vi "Validate Configuration Metadata.vi"(8 "error in (no error)":errorcluster, 11 "MeasurementPluginService in":refnum<class "MeasurementPluginService.lvclass">) -> (0 "error out":errorcluster, 3 "MeasurementPluginService out":refnum<class "MeasurementPluginService.lvclass">)   [LabVIEW 2020, in "MeasurementLink Measurement Server.lvlib"]
uses:
  MeasurementLink Measurement Server.lvlib
  <vilib>/Utility/Data Type/NI_Data Type.lvlib
  Classes/MeasurementPluginService/MeasurementPluginService.lvclass
  Error Strings Global Internal.vi
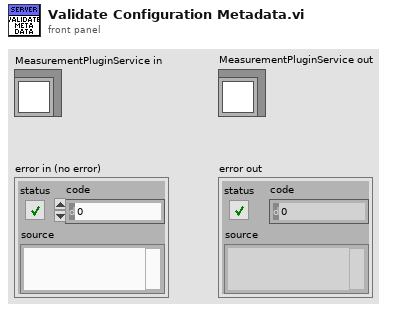
[diagram p1: front panel]
types:
  T1 = typedef "MeasurementLink Measurement Server.lvlib/MeasurementPluginService.lvclass/Plugin Paths.ctl" = cluster{"Get Measurement Details VI Path":path, "Get Type Specializations VI Path":path, "Get UI Details VI Path":path, "Measurement Logic VI Path":path, "Measurement Configuration CTL Path":path, "Measurement Results CTL Path":path}
  T2 = typedef "MeasurementLink Measurement Server.lvlib/Parameter Type Specialization.ctl" = cluster{"Parameter Name":string, "Type Specialization":T3, "Annotations":cluster{"Key":T4, "Value":string}[]}
  T3 = typedef "MeasurementLink Measurement Server.lvlib/Type Specialization.ctl" = enum16{"none", "pin", "path", "enum"}
  T4 = typedef "MeasurementLink Measurement Server.lvlib/Type Specialization Key.ctl" = enum16{"none", "pin.instrument_type", "enum.values"}
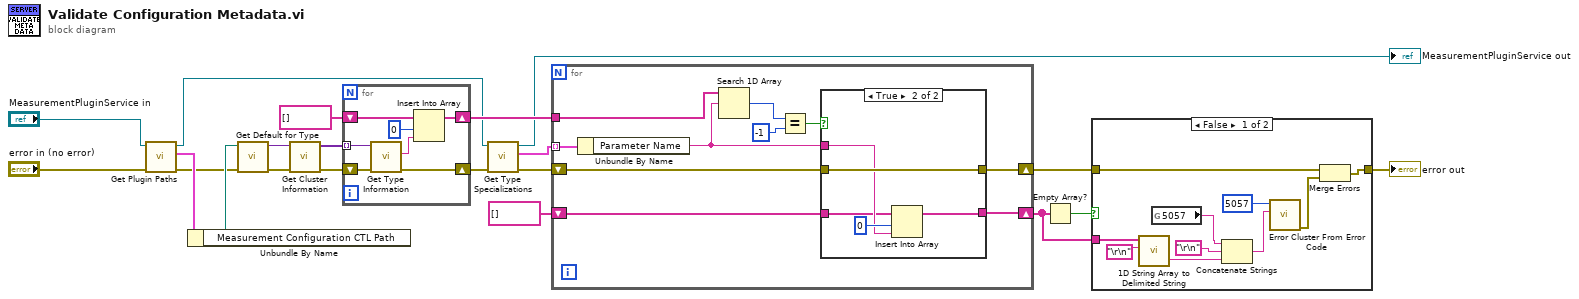
[diagram p0: block diagram]
diagram:
  n1 = call-dynamic "Get Plugin Paths.vi"("error in (no error)"="error in (no error)", "MeasurementPluginService in"="MeasurementPluginService in") -> ("error out"=w9:errorcluster, "Plugin Paths"=w11:T1, "MeasurementPluginService out"=w12:refnum<class "MeasurementPluginService.lvclass">)  [unwired: 7 in]
  n2 = Unbundle By Name(w11) -> ("Measurement Configuration CTL Path"=w10:path)
  n3 = call "Get Default for Type.vi"("error in (no error)"=w9, "Path of Type"=w10) -> ("error out"=w8:errorcluster, "Default for Type"=w17:variant)  [unwired: 8 in]
  n4 = call <vilib>:"Get Cluster Information.vi"("error in (no error)"=w8, "variant"=w17) -> ("error out"=w7:errorcluster, "cluster elements"=w21:variant[])  [unwired: 8 in]
  n5 = for {
    tunnel: w21 -> [w28] mode=indexing
    shift-right: [w24] -> w19
    shift-left: string[] [] -> [w26]
    shift-right: [w22] -> w6
    shift-left: w7 -> [w23]
    n6 = call <vilib>:"Get Type Information.vi"("error in (no error)"=w23, "variant"=w28) -> ("error out"=w22:errorcluster, "name"=w25:string)  [unwired: 5 in, 3 out]
    n7 = Insert Into Array(array=w26, index=0, new element=w25) -> (w24:string[])
  }
  n8 = call-dynamic "Get Type Specializations.vi"("error in (no error)"=w6, "MeasurementPluginService in"=w12) -> ("error out"=w16:errorcluster, "Type Specializations"=w15:T2[], "MeasurementPluginService out"=→"MeasurementPluginService out":refnum<class "MeasurementPluginService.lvclass">)  [unwired: 7 in]
  n9 = for {
    tunnel: w15 -> [w38] mode=indexing
    shift-right: [w32] -> w2
    shift-left: w16 -> [w33]
    tunnel: w19 -> [w37]
    shift-right: [w29] -> w5
    shift-left: string[] [] -> [w31]
    n10 = Unbundle By Name(w38) -> ("Parameter Name"=w30:string)
    n11 = Search 1D Array(1D array=w37, element=w30) -> (index of element=w36:i32)  [unwired: 1 in]
    n12 = Equal?(x=w36, y=-1) -> (x = y?=w34:bool)
    n13 = case shown="True" w34 {
      tunnel: w33 -> [w40 w45]
      tunnel: [w40 w45] -> w32
      tunnel: w31 -> [w39 w42]
      tunnel: w30 -> [_ w43]
      tunnel: [w39 w41] -> w29
      frame False {
      }
      frame True {
        n14 = Insert Into Array(array=w42, index=0, new element=w43) -> (w41:string[])
      }
    }
  }
  n15 = Empty Array?(array=w5) -> (empty?=w4:bool)
  n16 = case shown="False" w4 {
    tunnel: w5 -> [w52 _]
    tunnel: w2 -> [w47 w56]
    tunnel: [w48 w56] -> w1
    frame False {
      n17 = call <vilib>:"1D String Array to Delimited String.vi"("delimiter"="\r\n", "string array"=w52) -> ("delimited string"=w53:string)  [unwired: 9 in]
      n18 = global read "Error Strings Global Internal.vi" "5057"() -> (w51:string)
      n19 = Concatenate Strings(w51, "\r\n", w53) -> (w49:string)
      n20 = call <vilib>:"Error Cluster From Error Code.vi"("error message (\"\")"=w49, "error code (0)"=5057) -> ("error out"=w46:errorcluster)  [unwired: 7 in]
      n21 = Merge Errors(w47, w46) -> (w48:errorcluster)
    }
    frame True {
    }
  }
  "error out" <- w1
